vi "TMDSinterpolater.vi"() -> ()   [LabVIEW 2016]
panel:
  out "XY Graph":cluster{"Y":dbl[], "Y":dbl[]}[](graph)
  in  "dt":dbl=1e-06 format="%#_6p"
  in  "Channels":string[](array[string])=["Field_fixed", "Vxx", "Vxy", "I"]
  in  "Path":path=path "\\\\Mac\\Home/Desktop/USB/122016/s012_122016.tdms"
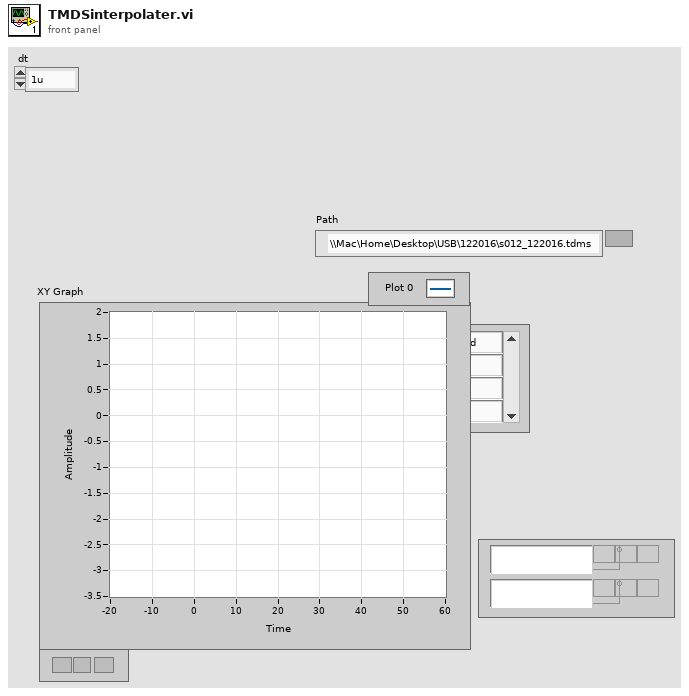
[diagram p1: front panel]
types:
  T1 = enum16{"open", "open or create", "create or replace", "create", "open (read-only)"}
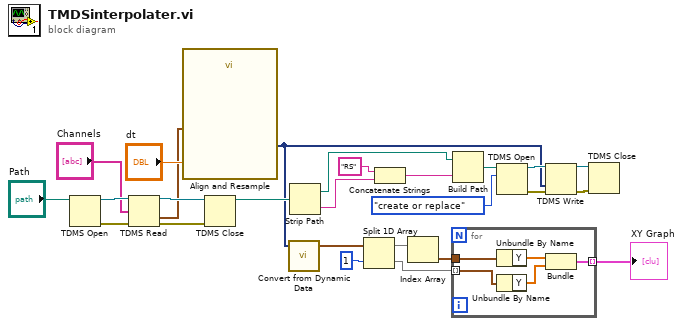
[diagram p0: block diagram]
diagram:
  n1 = TDMS Open(11:"Path") -> (0:w25:errorcluster, 3:w26:refnum<k34>)  [unwired: 6 in]
  n2 = TDMS Read(0:w26, 7:"Channels", 11:w25) -> (4:w24:refnum<k34>, 10:w19:waveform(dbl)[], 15:w23:errorcluster)  [unwired: 5 in, 3 out]
  n3 = call "Align and Resample"("dt"="dt", "Signals"=w19) -> ("Resampled Signals"=w2:dynamicdata)  [unwired: 7 in, 2 out]
  n4 = TDMS Close(8:w23, 11:w24) -> (3:w12:path)  [unwired: 1 out]
  n5 = call "Convert from Dynamic Data"("Dynamic Data Type"=w2) -> ("Array of Waveform"=w18:waveform(dbl)[])  [unwired: 3 in]
  n6 = Strip Path(path=w12) -> (stripped path=w9:path, name=w11:string)
  n7 = Split 1D Array(array=w18, index=1) -> (first subarray=w16:waveform(dbl)[], second subarray=w15:waveform(dbl)[])
  n8 = Concatenate Strings("RS" ("string"), w11) -> (w8:string)
  n9 = Index Array(array=w16) -> (element=w13:waveform(dbl))  [unwired: 1 in]
  n10 = for {
    tunnel: w13 -> [w31]
    tunnel: w15 -> [w30] mode=indexing
    tunnel: [w29] -> w14 mode=indexing
    n11 = Unbundle By Name(w31) -> ("Y"=w28:dbl[])
    n12 = Unbundle By Name(w30) -> ("Y"=w27:dbl[])
    n13 = Bundle("Y"=w28, "Y"=w27) -> (w29:cluster{"Y":dbl[], "Y":dbl[]})  [unwired: 1 in]
  }
  "XY Graph" <- w14
  n14 = Build Path(base path=w9, name or relative path=w8) -> (appended path=w3:path)
  n15 = TDMS Open(10:T1."create or replace" ("operation (0:open)"), 11:w3) -> (0:w6:errorcluster, 3:w7:refnum<k34>)  [unwired: 5 in]
  n16 = TDMS Write(0:w7, 9:w2, 11:w6) -> (4:w5:refnum<k34>, 15:w4:errorcluster)  [unwired: 3 in, 2 out]
  n17 = TDMS Close(8:w4, 11:w5) -> ()  [unwired: 2 out]
